vi "eeprom.vi"() -> ()   [LabVIEW 2017]
panel:
  out "length":i32
  out "data string":string
  out "Value out":string
  out "value":u32
  in  "number":u32
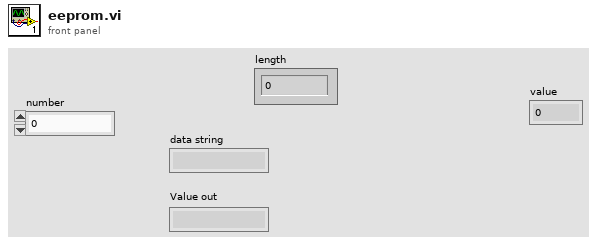
[diagram p1: front panel]
types:
  T1 = enum16{"big-endian, network order", "native, host order", "little-endian"}
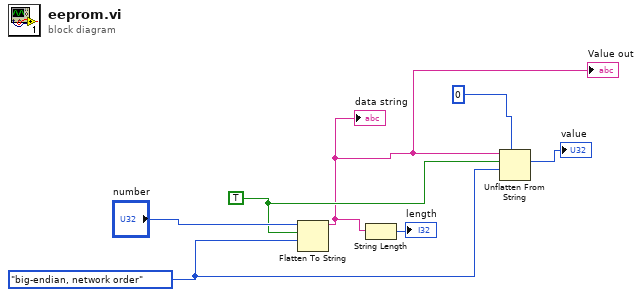
[diagram p0: block diagram]
diagram:
  w4 = T1."big-endian, network order" ("byte order (0:big-endian, network order)")
  w3 = TRUE ("prepend array or string size? (T)")
  n1 = Flatten To String(anything="number", prepend array or string size? (T)=w3, byte order (0:big-endian, network order)=w4) -> (data string=w2:string)  [unwired: 1 in, 2 out]
  "Value out" <- w2
  "data string" <- w2
  n2 = String Length(string=w2) -> (length=→"length":i32)
  n3 = Unflatten From String(type=u32 0, binary string=w2, data includes array or string size? (T)=w3, byte order (0:big-endian, network order)=w4) -> (value=→"value":u32)  [unwired: 1 in, 2 out]
